vi "Drive Base Controller.vi"(8 "error in":errorcluster) -> ()   [LabVIEW 2019]
doc: "This VI executes continuously carrying out the current operation and responding to updates or new operations. It will often contain the timing or control code that is difficult to place directly in TeleOp. This VI generally opens all sensors and motors and isolates the rest of the robot code from knowing how the operations are carried out."
uses:
  <vilib>/Rock Robotics/WPI/Framework/Completion Status.ctl
  Drive Base Setpoints.ctl
  Drive Base Operations.ctl
  <vilib>/Rock Robotics/WPI/ThirdParty/REV Robotics/SPARK MAX/Typedef/Spark MAX Control Type.ctl
  <vilib>/Rock Robotics/Network Tables/NT Write Boolean.vi
panel:
  in  "Interactive Values":T1
  out "Current\nCmd":string
  in  "Buttons":cluster{"Execute Cmd":bool, "Abort Cmd":bool}
  out "Command Timing":cluster{"Start Time (ms)":u32, "Iterations":i32}
  out "Status":T3
  # "Tip: It may be helpful to observe inputs and sensor values.\nYou may also want to display tuning or debugging controls."
  # "Interactive Command: You may fill in the settings for a command\nand schedule it with the Execute button. You can observe and abort\nany command while fine tuning the code for the controller."
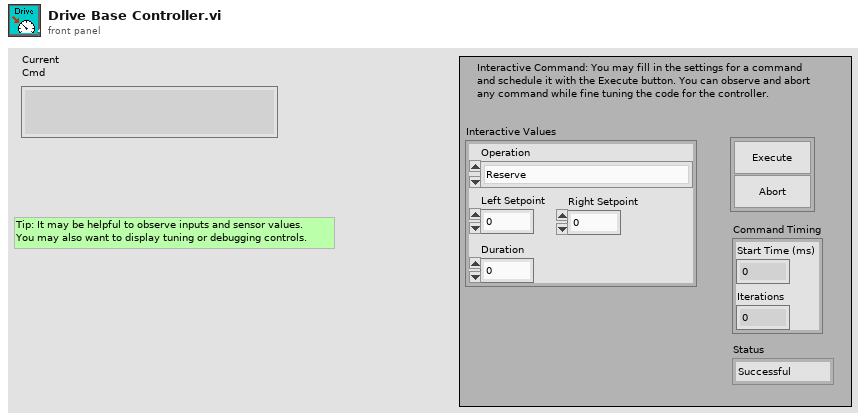
[diagram p1: front panel]
types:
  T1 = typedef "Drive Base Setpoints.ctl" = cluster{"Operation":T2, "Left Setpoint":dbl, "Duration":dbl, "Right Setpoint":dbl}
  T2 = typedef "Drive Base Operations.ctl" = enum16{"Reserve", "Read Current", "Immediate"}
  T3 = typedef "Completion Status.ctl" = enum16{"Successful", "Aborted", "Incomplete"}
  T4 = typedef "WPI_MotorControlDeviceRef.ctl" = cluster{"DeviceStatus":errorcluster, "Type":T5, "PWM":cluster{"PWM Channel":T6, "DeadBand":T7}, "CAN":cluster{"Device Number":u8, "SetOutput VI Ref":variant, "GetOutput VI Ref":variant, "Enable VI Ref":variant, "Disable VI Ref":variant, "Data":variant}, "Invert":bool, "DIO PWM":cluster{"PWM \"Enable\" Channel":T6, "DIOChannel":T8, "PWM Rate":dbl}}
  T5 = typedef "WPI_MotorControlType.ctl" = enum16{"PWM", "CAN", "DIO PWM"}
  T6 = typedef "FPGA_DIOPWMChannel.ctl" = enum8{"PWM 0", "PWM 1", "PWM 2", "PWM 3", "PWM 4", "PWM 5", "PWM 6", "PWM 7", "PWM 8", "PWM 9", "PWM MXP 0", "PWM MXP 1", "PWM MXP 2", "PWM MXP 3", "PWM MXP 4", "PWM MXP 5", "PWM MXP 6", "PWM MXP 7", "PWM MXP 8", "PWM MXP 9", "Invalid"}
  T7 = typedef "WPI_PWMDeadband.ctl" = cluster{"Name":string, "maxPositivePwm":i32, "minPositivePwm":i32, "centerPwm":i32, "maxNegativePwm":i32, "minNegativePwm":i32, "angularRange":u16}
  T8 = typedef "FPGA_DIOChannel.ctl" = enum8{"DIO 0", "DIO 1", "DIO 2", "DIO 3", "DIO 4", "DIO 5", "DIO 6", "DIO 7", "DIO 8", "DIO 9", "DIO MXP 0", "DIO MXP 1", "DIO MXP 2", "DIO MXP 3", "DIO MXP 4", "DIO MXP 5", "DIO MXP 6", "DIO MXP 7", "DIO MXP 8", "DIO MXP 9", "DIO MXP 10", "DIO MXP 11", "DIO MXP 12", "DIO MXP 13", "DIO MXP 14", "DIO MXP 15", "SPI Port CS1", "SPI Port CS2", "SPI Port CS3", "SPI Port MISO", "SPI Port MOSI", "Invalid"}
  T9 = typedef "Command Status Info.ctl" = cluster{"Name":string, "Status":T3, "notifier out":T10}
  T10 = typedef "Completion Notifier.ctl" = refnum<notifier>
  T11 = cluster{"Current Command":T1, "Command Timing":cluster{"Start Time (ms)":u32, "Iterations":i32}, "Command Arguments":cluster{"Command Info":T9, "Description":string, "Default Command":T1, "queue out":refnum<queue>, "Subsystem Name":string}}
  T12 = typedef "Spark MAX Control Type.ctl" = enum16{"Percent VBus", "Voltage", "Velocity", "Position", "Smart Motion", "Current", "Smart Velocity"}
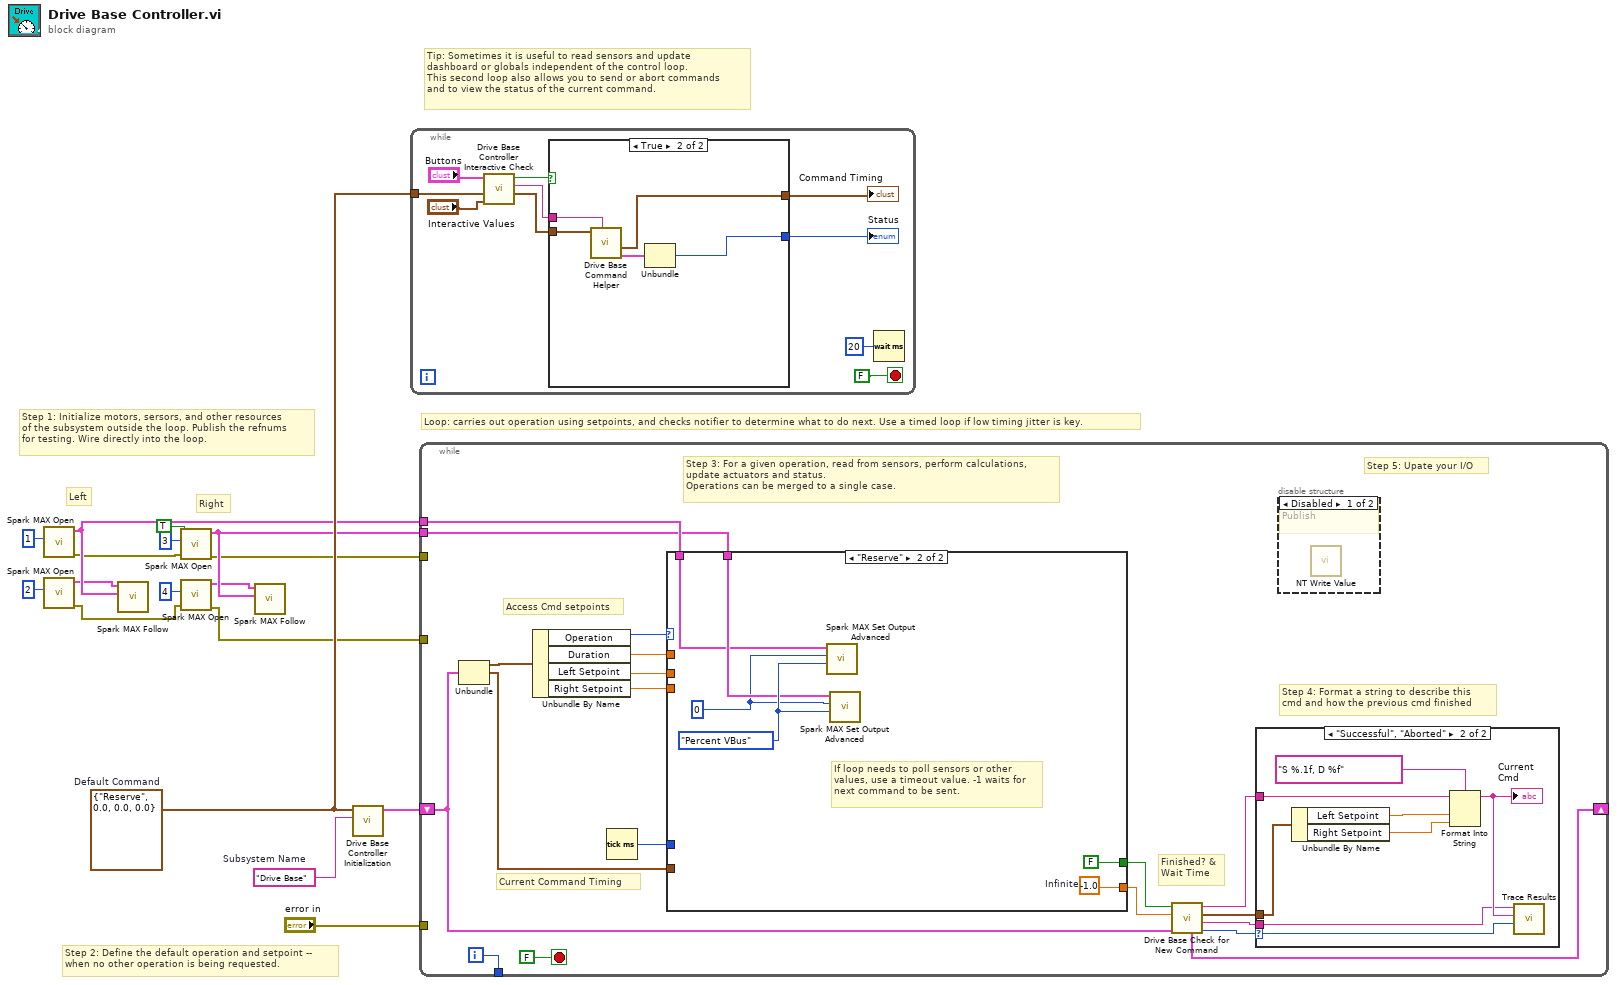
[diagram p0: block diagram]
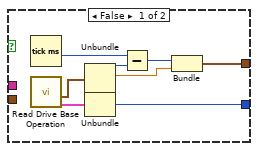
[diagram p2: hidden frame]
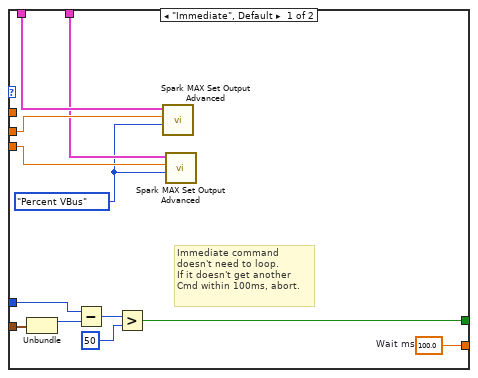
[diagram p5: hidden frame]
diagram:
  w14 = T1 {"Operation"=enum."Reserve", "Left Setpoint"=0.0, "Duration"=0.0, "Right Setpoint"=0.0}  # Default Command
  w15 = "Drive Base"  # Subsystem Name
  # "Right"
  # "Left"
  # "Tip: Sometimes it is useful to read sensors and update\ndashboard or globals independent of the control loop.\nThis second loop also allows you to send or abort commands\nand to view the status of the current command."
  # "Step 2: Define the default operation and setpoint --\nwhen no other operation is being requested."
  # "Step 1: Initialize motors, sersors, and other resources\nof the subsystem outside the loop. Publish the refnums\nfor testing. Wire directly into the loop."
  # "Loop: carries out operation using setpoints, and checks notifier to determine what to do next. Use a timed loop if low timing jitter is key."
  n1 = call <vilib>:"Spark MAX Open.vi"("Device Number"=u8 1) -> ("error out"=w10:errorcluster, "MotorControlDeviceRef"=w12:T4)  [unwired: 9 in]
  n2 = call <vilib>:"Spark MAX Open.vi"("Device Number"=u8 2) -> ("error out"=w3:errorcluster, "MotorControlDeviceRef"=w6:T4)  [unwired: 9 in]
  n3 = call <vilib>:"Spark MAX Follow.vi"("Master Controller"=w12, "MotorControlDeviceRef"=w6) -> ()  [unwired: 8 in, 2 out]
  n4 = call <vilib>:"Spark MAX Open.vi"("error in (no error)"=w10, "Invert"=TRUE, "Device Number"=u8 3) -> ("error out"=w9:errorcluster, "MotorControlDeviceRef"=w11:T4)  [unwired: 7 in]
  n5 = call <vilib>:"Spark MAX Open.vi"("error in (no error)"=w3, "Device Number"=u8 4) -> ("error out"=w8:errorcluster, "MotorControlDeviceRef"=w7:T4)  [unwired: 8 in]
  n6 = call <vilib>:"Spark MAX Follow.vi"("Master Controller"=w11, "MotorControlDeviceRef"=w7) -> ()  [unwired: 8 in, 2 out]
  n7 = call "Drive Base Controller Initialization.vi"("Subsystem Name"=w15, "Default Command"=w14) -> ("Current Command"=w16:T11)  [unwired: 9 in]
  n8 = while {
    tunnel: w14 -> [w24]
    stop <- FALSE stop-if-true
    n9 = call "Drive Base Controller Interactive Check.vi"("Interactive Command in"="Interactive Values", "Default Command"=w24, "Buttons"="Buttons") -> ("Interactive Command out"=w21:T1, "Trace String"=w22:string, "Schedule"=w23:bool)  [unwired: 6 in]
    n10 = case shown="True" w23 {
      tunnel: [w35 w40] -> w20
      tunnel: w21 -> [_ w38]
      tunnel: [w31 w36] -> w19
      tunnel: w22 -> [_ w39]
      frame False {
        n11 = Tick Count (ms)() -> (millisecond timer value=w30:u32)
        n12 = call "Read Drive Base Operation.vi"() -> ("Command Info"=w28:T9, "SubSystem Data"=w29:T1)  [unwired: 9 in, 1 out]
        n13 = Unbundle(w29) -> ("Operation"=w34:T2, "Left Setpoint"=w32:dbl)  [unwired: 2 out]
        n14 = Unbundle(w28) -> ("Status"=w35:T3)  [unwired: 2 out]
        n15 = Subtract(x=w30, y=w34) -> (x-y=w33:u32)
        n16 = Bundle(w33, "Left Setpoint"=w32) -> (w31:cluster{u32, "Left Setpoint":dbl})  [unwired: 1 in]
      }
      frame True {
        n17 = call "Drive Base Command Helper.vi"("Description"=w39, "SubSystem Data"=w38) -> ("Command Info Out"=w37:T9, "Command Timing"=w36:cluster{"Start Time (ms)":u32, "Iterations":i32})  [unwired: 7 in, 1 out]
        n18 = Unbundle(w37) -> ("Status"=w40:T3)  [unwired: 2 out]
      }
    }
    "Status" <- w20
    "Command Timing" <- w19
    n19 = Wait (ms)(milliseconds to wait=u32 20) -> ()  [unwired: 1 out]
  }
  n20 = while {
    shift-right: [w51] -> _
    shift-left: w16 -> [w44]
    tunnel: [w58] -> _
    tunnel: "error in" -> [_]
    tunnel: w12 -> [w42]
    tunnel: w11 -> [w41]
    tunnel: w9 -> [_]
    tunnel: w8 -> [_]
    i -> [w58]
    stop <- FALSE stop-if-true
    # "Step 5: Upate your I/O"
    # "Step 4: Format a string to describe this\ncmd and how the previous cmd finished"
    # "Current Command Timing"
    # "Access Cmd setpoints"
    # "Finished? &\nWait Time"
    # "Step 3: For a given operation, read from sensors, perform calculations,\nupdate actuators and status.\nOperations can be merged to a single case."
    n21 = Unbundle(w44) -> ("Current Command"=w57:T1, "Command Timing"=w53:cluster{"Start Time (ms)":u32, "Iterations":i32})  [unwired: 1 out]
    n22 = Unbundle By Name(w57) -> ("Operation"=w56:T2, "Duration"=w55:dbl, "Left Setpoint"=w52:dbl, "Right Setpoint"=w43:dbl)
    n23 = Tick Count (ms)() -> (millisecond timer value=w54:u32)
    n24 = case shown="\"Reserve\"" w56 {
      tunnel: [w79 w85] -> w49
      tunnel: [w73 FALSE ("ignore previous (F)")] -> w50
      tunnel: w53 -> [w75 _]
      tunnel: w55 -> [_ _]
      tunnel: w54 -> [w74 _]
      tunnel: w52 -> [w72 _]
      tunnel: w43 -> [w71 _]
      tunnel: w42 -> [w70 w81]
      tunnel: w41 -> [w69 w82]
      frame "Immediate", Default {
        w68 = Spark_MAX_Control_Type."Percent VBus" ("Control Mode")
        w79 = 100.0  # Wait ms
        # "Immediate command\ndoesn't need to loop.\nIf it doesn't get another\nCmd within 100ms, abort."
        n25 = Unbundle(w75) -> ("Start Time (ms)"=w78:u32)  [unwired: 1 out]
        n26 = Subtract(x=w74, y=w78) -> (x-y=w77:u32)
        n27 = Greater?(x=w77, y=u8 50 ("Left Motor")) -> (0:w73:bool)
        n28 = call <vilib>:"Spark MAX Set Output Advanced.vi"("Control Mode"=w68, "Setpoint"=w72, "MotorControlDevRef"=w70) -> ()  [unwired: 7 in, 2 out]
        n29 = call <vilib>:"Spark MAX Set Output Advanced.vi"("Control Mode"=w68, "Setpoint"=w71, "MotorControlDevRef"=w69) -> ()  [unwired: 7 in, 2 out]
      }
      frame "Reserve" {
        w80 = 0
        w83 = Spark_MAX_Control_Type."Percent VBus" ("Control Mode")
        w85 = -1.0  # Infinite
        # "If loop needs to poll sensors or other\nvalues, use a timeout value. -1 waits for\nnext command to be sent."
        n30 = call <vilib>:"Spark MAX Set Output Advanced.vi"("Control Mode"=w83, "Setpoint"=w80, "MotorControlDevRef"=w81) -> ()  [unwired: 7 in, 2 out]
        n31 = call <vilib>:"Spark MAX Set Output Advanced.vi"("Control Mode"=w83, "Setpoint"=w80, "MotorControlDevRef"=w82) -> ()  [unwired: 7 in, 2 out]
      }
    }
    n32 = call "Drive Base Check for New Command.vi"("Current Command"=w44, "Wait time (ms)"=w49, "Finished?"=w50) -> ("Completion"=w45:T3, "Subsystem Name"=w46:string, "Current Command"=w47:T1, "Initial Trace String"=w48:string, "NextCommand"=w51:T11)  [unwired: 4 in]
    n33 = case shown="\"Successful\", \"Aborted\"" w45 {
      selector: w45 -> [_ w67]
      tunnel: w48 -> [_ w63]
      tunnel: w47 -> [_ w64]
      tunnel: w46 -> [_ w60]
      frame "Incomplete", Default {
        # "Continuing current command"
      }
      frame "Successful", "Aborted" {
        # "Report and setup for next command"
        n34 = Unbundle By Name(w64) -> ("Left Setpoint"=w66:dbl, "Right Setpoint"=w61:dbl)
        n35 = Format Into String(format string="S %.1f, D %f", initial string=w63, w66, w61) -> (resulting string=w62:string)  [unwired: 1 in, 1 out]
        "Current\nCmd" <- w62
        n36 = call <vilib>:"Trace Results.vi"("Status of previous command"=w67, "Description"=w62, "Subsystem"=w60) -> ()  [unwired: 9 in]
      }
    }
    n37 = disable-structure shown="Disabled" {
      frame Disabled {
        # "Publish"
        n38 = call-poly <vilib>:"NT Write Value.vi"() -> ()  [unwired: 11 in, 1 out]
      }
      frame Enabled {
      }
    }
  }
